vi "GetWindowBordersSize.vi"(8 "No Error":errorcluster, 11 "Window [SDL_Window *]":i64) -> (0 "Error Out":errorcluster, 1 "Right":i32, 2 "Bottom":i32, 3 "Left":i32, 5 "Top":i32)   [LabVIEW 2024, in "SDL3.lvlib" / "Video.lvlib"]
doc: "<B>Summary</B>\nGet the size of a window's borders (decorations) around the client area.\n\n<B>Remarks</B>\nNote: If this function fails (returns false), the size values will be initialized to 0, 0, 0, 0, as if the window in question was borderless.\n\nNote: This function may fail on systems where the window has not yet been decorated by the display server (for example, immediately after calling SDL_CreateWindow). It is recommended that you wait at least until the window has been presented and composited, so that the window system has a chance to decorate the window and provide the border dimensions to SDL.\n\nThis function also returns false if getting the information is not supported."
uses:
  Video.lvlib
  Error/Error.lvlib
  Lib/SDL3-32.dll
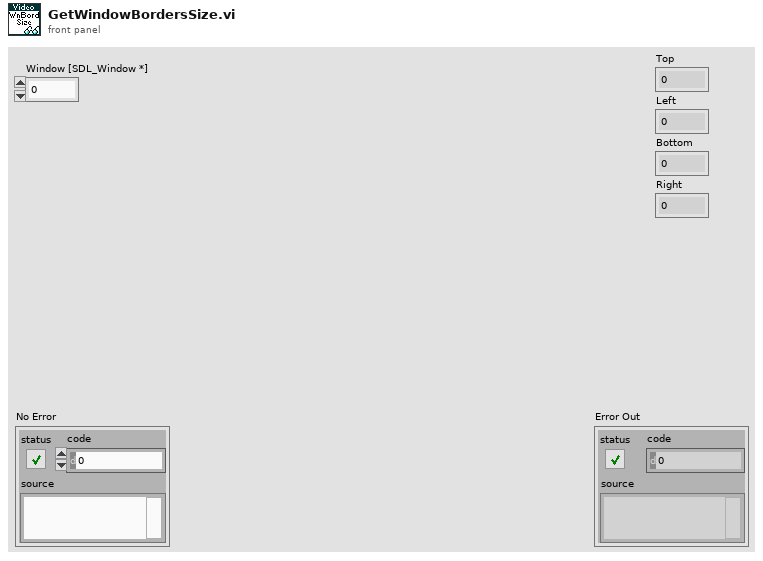
[diagram p1: front panel]
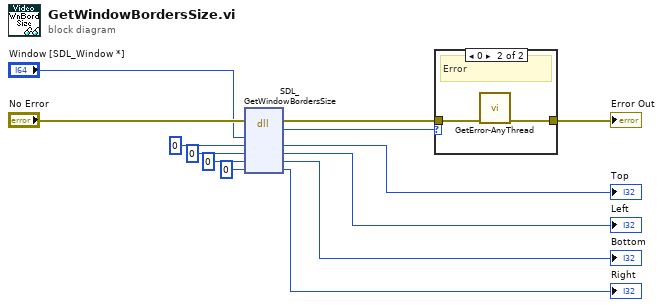
[diagram p0: block diagram]
diagram:
  n1 = dll-call lib="C:/Users/Thomas/Documents/Projects/LV-SDL3/Lib/SDL3-*.*" fn="SDL_GetWindowBordersSize"(error in="No Error", "window"="Window [SDL_Window *]", "top"=0, "left"=0, "bottom"=0, "right"=0) -> (error out=w6:errorcluster, "return type"=w5:i32, "top"=→"Top":i32, "left"=→"Left":i32, "bottom"=→"Bottom":i32, "right"=→"Right":i32)  [unwired: 3 in, 1 out]
  n2 = case shown="0" w5 {
    tunnel: w6 -> [w14 w16]
    tunnel: [w14 w15] -> w12
    frame Default {
      # "Ok"
    }
    frame 0 {
      # "Error"
      n3 = call "GetError-AnyThread.vi"("No Error"=w16) -> ("Error Out"=w15:errorcluster)  [unwired: 10 in]
    }
  }
  "Error Out" <- w12
